vi "Endpoint.vi"(1 "timeout in ms (-1)":i32=-1, 5 "is valid (T)":bool=TRUE, 7 "element in":T1, 9 "size (0)":i32, 11 "is last element (F)":bool, 12 "abort (F)":bool) -> (3 "timed out?":bool, 4 "channel out":T2, 13 "count":i32, 14 "aborted?":bool)   [LabVIEW 2017, in "Stream-t'WPI_EncoderType.ctl'.lvlib"]
uses:
  <extravilib>/ChannelInstances/Stream-t'WPI_EncoderType.ctl'.lvlib
  <extravilib>/ChannelInstances/Stream-t'WPI_EncoderType.ctl'/)Channel.ctl
  <vilib>/Rock Robotics/WPI/Encoder/WPI_EncoderType.ctl
  <extravilib>/ChannelInstances/Stream-t'WPI_EncoderType.ctl'/ChannelOp.ctl
  <resource>/ChannelSupport/_ChannelSupport/_ChannelSupport.lvlib
panel:
  # "legal combinations:\n\n    abort\n    timedout\n    valid\n    valid, last element\n    last element"
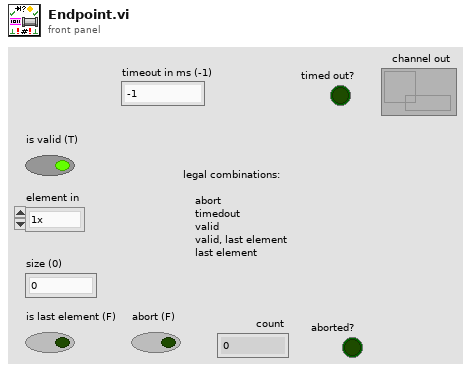
[diagram p1: front panel]
types:
  T1 = typedef "WPI_EncoderType.ctl" = enum16{"1x", "2x", "4x"}
  T2 = typedef "Stream-t'WPI_EncoderType.ctl'.lvlib/)Channel.ctl" = refnum<queue>
  T3 = typedef "Stream-t'WPI_EncoderType.ctl'.lvlib/ChannelOp.ctl" = enum16{"init", "write", "read", "probe"}
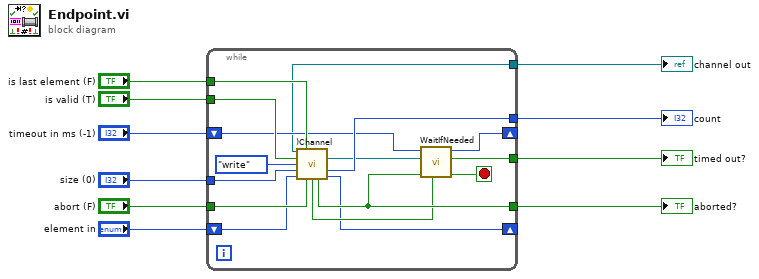
[diagram p0: block diagram]
diagram:
  n1 = while {
    tunnel: [w19] -> w9
    tunnel: [w15] -> w8
    tunnel: [w26] -> w7
    tunnel: "abort (F)" -> [w25]
    tunnel: "size (0)" -> [w23]
    tunnel: "is last element (F)" -> [w21]
    tunnel: "is valid (T)" -> [w20]
    shift-right: [w14] -> _
    shift-left: "timeout in ms (-1)" -> [w17]
    shift-right: [w12] -> _
    shift-left: "element in" -> [w22]
    tunnel: "channel out" -> [w11]
    stop <- w16 stop-if-true
    n2 = call <extravilib>:")Channel.vi"("last element in"=w21, "valid"=w20, "channelOp"=ChannelOp."write", "size"=w23, "element in"=w22, "abort in"=w25) -> ("channel in"=w11:T2, "wait"=w18:refnum<k4>, "count"=w26:i32, "retry"=w13:bool, "aborted"=w19:bool, "element out"=w12:T1)  [unwired: 1 in, 3 out]
    n3 = call <resource>:"WaitIfNeeded.vi"("retry"=w13, "stopping"=w19, "wait"=w18, "_timeout (ms) in"=w17) -> ("stop loop"=w16:bool, "timed out"=w15:bool, "_timeout (ms) out"=w14:i32)  [unwired: 5 in]
  }
  "count" <- w7
  "timed out?" <- w8
  "aborted?" <- w9
